vi "Trapezoidal SetAngle V2.vi"(0 "Current Angle":dbl, 5 "Desired Angle":dbl, 7 "\"dashboard values\"":T1) -> (1 "State":string, 2 "Completed?":bool, 3 "W reach in use":bool, 4 "Angular Velocity":dbl, 6 "Angular Acceleration":dbl, 8 "Current Angle":dbl, 10 "Time Completed":dbl, 13 "Reachable Velocity":dbl, 14 "Area":dbl, 15 "Times":cluster{"ta":dbl, "tc":dbl, "tf":dbl})   [LabVIEW 2015]
uses:
  TrapModeSetAngle.ctl
  Change Detect Double.vi
  Change Detect Int.vi
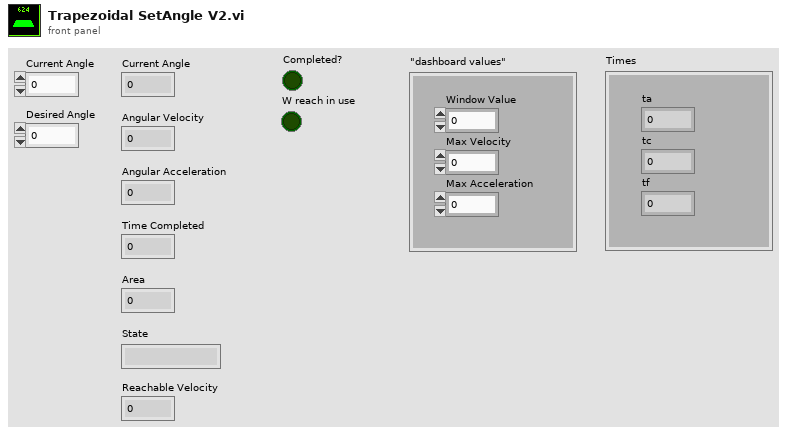
[diagram p1: front panel]
types:
  T1 = cluster{"Window Value":dbl, "Max Velocity":dbl, "Max Acceleration":dbl}
  T2 = typedef "TrapModeSetAngle.ctl" = enum16{"Accelerate", "Decelerate", "Cruz", "Finish"}
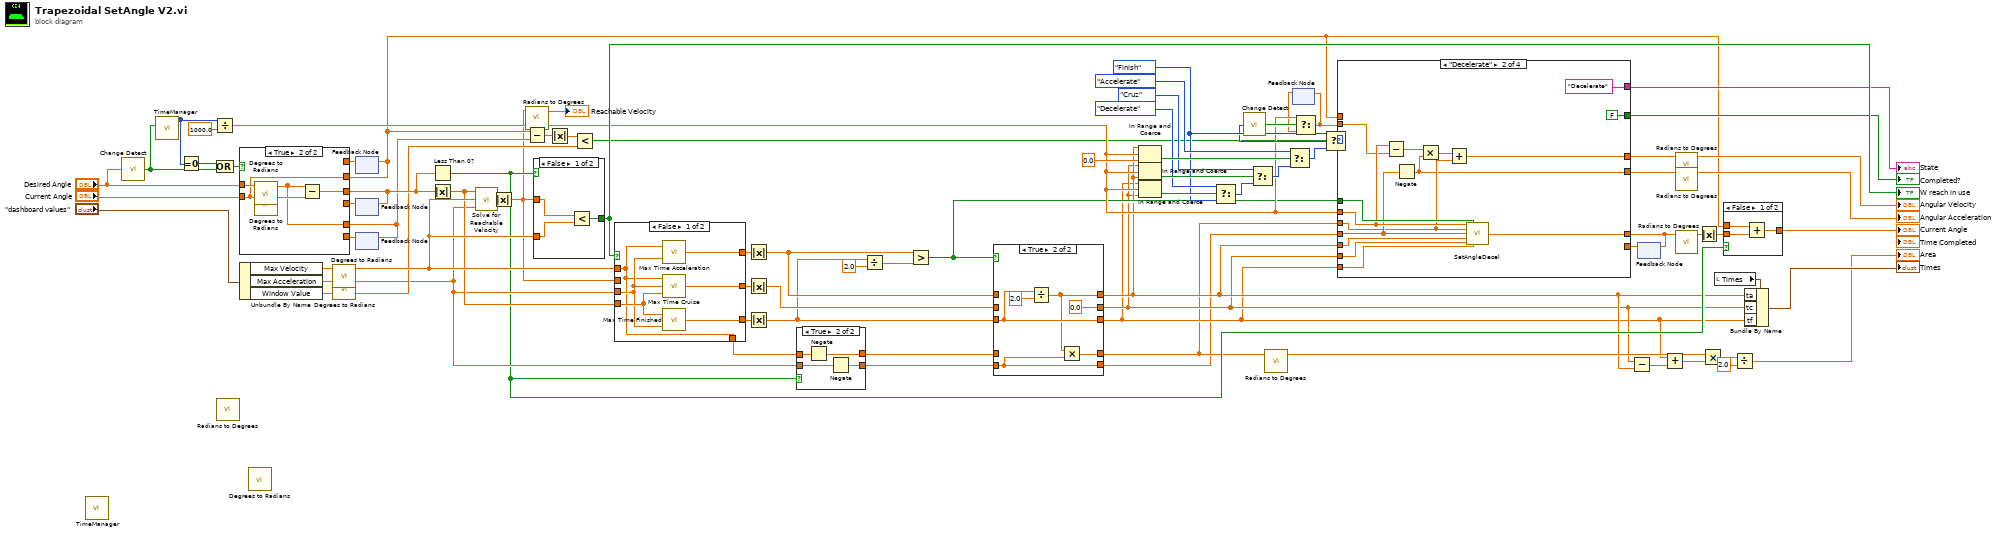
[diagram p0: block diagram]
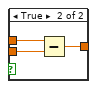
[diagram p3: hidden frame]
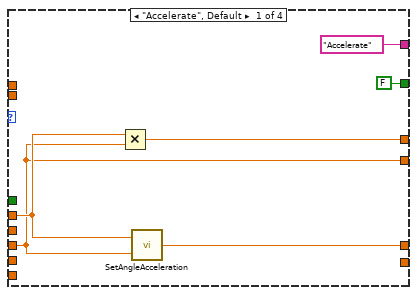
[diagram p5: hidden frame]
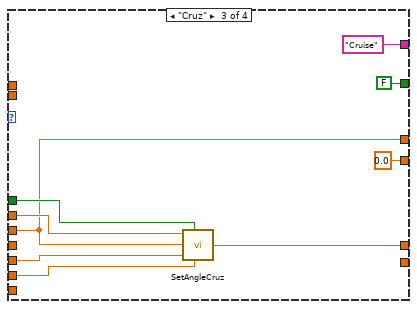
[diagram p6: hidden frame]
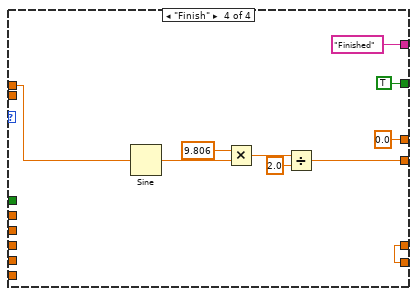
[diagram p7: hidden frame]
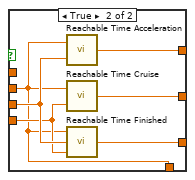
[diagram p8: hidden frame]
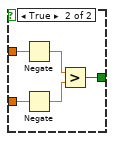
[diagram p9: hidden frame]
diagram:
  w54 = TrapModeSetAngle."Finish" ("Mode")
  n1 = call "TimeManager.vi"() -> ()  [unwired: 10 in, 2 out]
  n2 = call-poly "Change Detect.vi"("In"="Desired Angle") -> ("Changed?"=w75:bool)
  n3 = call "TimeManager.vi"("Reset?"=w75) -> ("Time Since Reset"=w65:u32)  [unwired: 9 in, 1 out]
  n4 = Equal To 0?(x=w65) -> (x = 0?=w74:bool)
  n5 = Divide(x=w65, y=1000.0) -> (x/y=w35:dbl)
  n6 = Compound Arithmetic op=OR(w74, w75) -> (w76:bool)
  n7 = call "Radians to Degrees.vi"() -> ()  [unwired: 5 in, 1 out]
  n8 = Unbundle By Name("\"dashboard values\"") -> ("Max Velocity"=w72:dbl, "Max Acceleration"=w71:dbl, "Window Value"=w49:dbl)
  n9 = call "Degrees to Radians.vi"() -> ()  [unwired: 5 in, 1 out]
  n10 = call "Degrees to Radians.vi"("Degrees IN"=w72) -> ("Radians OUT"=w70:dbl)  [unwired: 4 in]
  n11 = call "Degrees to Radians.vi"("Degrees IN"=w71) -> ("Radians OUT"=w47:dbl)  [unwired: 4 in]
  n12 = feedback #1() -> (w77:dbl)  [unwired: 1 in]
  n13 = feedback #2() -> (w78:dbl)  [unwired: 1 in]
  n14 = feedback #3() -> (w53:dbl)  [unwired: 1 in]
  n15 = case shown="True" w76 {
    tunnel: "Desired Angle" -> [_ w88]
    tunnel: "Current Angle" -> [_ w84]
    tunnel: [w83 w87] -> w73
    tunnel: w78 -> [w83 _]
    tunnel: [w82 w84] -> w24
    tunnel: w77 -> [w82 _]
    tunnel: [w81 w85] -> w52
    tunnel: w53 -> [w81 _]
    frame False {
    }
    frame True {
      n16 = call "Degrees to Radians.vi"("Degrees IN"=w88) -> ("Radians OUT"=w85:dbl)  [unwired: 4 in]
      n17 = call "Degrees to Radians.vi"("Degrees IN"=w84) -> ("Radians OUT"=w86:dbl)  [unwired: 4 in]
      n18 = Subtract(x=w85, y=w86) -> (x-y=w87:dbl)
    }
  }
  n19 = feedback-in #1(w24) -> ()
  n20 = feedback-in #2(w73) -> ()
  n21 = feedback-in #3(w52) -> ()
  n22 = Less Than 0?(x=w73) -> (x < 0?=w41:bool)
  n23 = Absolute Value(x=w73) -> (abs(x)=w69:dbl)
  n24 = call "Solve for Reachable Velocity.vi"("Max Acceleration"=w47, "Max Velocity"=w70, "Angular Displacement"=w69) -> ("Reachable Velocity"=w22:dbl)
  n25 = Absolute Value(x=w22) -> (abs(x)=w8:dbl)
  n26 = call "Radians to Degrees.vi"("Radians"=w8) -> ("Degrees"=→"Reachable Velocity":dbl)  [unwired: 4 in]
  n27 = Subtract(x=w24, y=w52) -> (x-y=w51:dbl)
  n28 = case shown="False" w41 {
    tunnel: w8 -> [w91 w96]
    tunnel: w70 -> [w90 w95]
    tunnel: [w89 w92] -> w42
    frame False {
      n29 = Less?(x=w91, y=w90) -> (x < y?=w89:bool)
    }
    frame True {
      n30 = Negate(x=w96) -> (-x=w94:dbl)
      n31 = Negate(x=w95) -> (-x=w93:dbl)
      n32 = Greater?(x=w94, y=w93) -> (0:w92:bool)
    }
  }
  "W reach in use" <- w42
  n33 = Absolute Value(x=w51) -> (abs(x)=w50:dbl)
  n34 = Less?(x=w50, y=w49) -> (x < y?=w25:bool)
  n35 = case shown="False" w42 {
    tunnel: w70 -> [w97 _]
    tunnel: w8 -> [_ w103]
    tunnel: w47 -> [w101 w108]
    tunnel: w69 -> [w102 w107]
    tunnel: [w100 w106] -> w18
    tunnel: [w99 w105] -> w19
    tunnel: [w98 w104] -> w20
    tunnel: [w97 w103] -> w48
    frame False {
      n36 = call "Max Time Acceleration.vi"("Max Acceleration"=w101, "Max Velocity"=w97) -> ("Max Time Acceleration"=w100:dbl)
      n37 = call "Max Time Cruise.vi"("Angle Displacement"=w102, "Max Acceleration"=w101, "Max Velocity"=w97) -> ("Max Time Cruise"=w99:dbl)
      n38 = call "Max Time Finished.vi"("Max Acceleration"=w101, "Angle Displacement"=w102) -> ("Max Time Finished"=w98:dbl)
    }
    frame True {
      n39 = call "Reachable Time Acceleration.vi"("Max Acceleration"=w108, "Reachable Angular Velocity"=w103) -> ("Reachable Time Acceleration"=w106:dbl)
      n40 = call "Reachable Time Cruise.vi"("Angle Displacement"=w107, "Reachable Angular Velocity"=w103) -> ("Reachable Time Cruise"=w105:dbl)
      n41 = call "Reachable Time Finished.vi"("Angle Displacement"=w107, "Max Acceleration"=w108, "Reachable Angular Velocity"=w103) -> ("Reachable Time Finished"=w104:dbl)
    }
  }
  n42 = Absolute Value(x=w18) -> (abs(x)=w11:dbl)
  n43 = Absolute Value(x=w19) -> (abs(x)=w10:dbl)
  n44 = Absolute Value(x=w20) -> (abs(x)=w9:dbl)
  n45 = case shown="True" w41 {
    tunnel: w48 -> [w110 w114]
    tunnel: w47 -> [w109 w113]
    tunnel: [w110 w112] -> w4
    tunnel: [w109 w111] -> w2
    frame False {
    }
    frame True {
      n46 = Negate(x=w114) -> (-x=w112:dbl)
      n47 = Negate(x=w113) -> (-x=w111:dbl)
    }
  }
  n48 = Divide(x=w9, y=2.0) -> (x/y=w45:dbl)
  n49 = Greater?(x=w11, y=w45) -> (0:w21:bool)
  n50 = case shown="True" w21 {
    tunnel: [w119 w122] -> w7
    tunnel: [w118 0.0 ("Reachable Time Cruise")] -> w6
    tunnel: [w117 w125] -> w5
    tunnel: w11 -> [w119 _]
    tunnel: w10 -> [w118 _]
    tunnel: w9 -> [w117 w125]
    tunnel: w4 -> [w116 _]
    tunnel: [w116 w121] -> w3
    tunnel: w2 -> [w115 w120]
    tunnel: [w115 w120] -> w1
    frame False {
    }
    frame True {
      n51 = Divide(x=w125, y=2.0) -> (x/y=w122:dbl)
      n52 = Multiply(x=w122, y=w120) -> (x*y=w121:dbl)
    }
  }
  n53 = In Range and Coerce(upper limit=w7, x=w35, lower limit=0.0) -> (In Range?=w63:bool)  [unwired: 1 out]
  n54 = In Range and Coerce(upper limit=w6, x=w35, lower limit=w7) -> (In Range?=w62:bool)  [unwired: 1 out]
  n55 = In Range and Coerce(upper limit=w5, x=w35, lower limit=w6) -> (In Range?=w60:bool)  [unwired: 1 out]
  n56 = Select(t=TrapModeSetAngle."Decelerate" ("Mode"), s=w60, f=w54) -> (s? t:f=w59:T2)
  n57 = Select(t=TrapModeSetAngle."Cruz" ("Mode"), s=w62, f=w59) -> (s? t:f=w61:T2)
  n58 = call "Radians to Degrees.vi"("Radians"=w3) -> ("Degrees"=w12:dbl)  [unwired: 4 in]
  n59 = Select(t=TrapModeSetAngle."Accelerate" ("Mode"), s=w63, f=w61) -> (s? t:f=w58:T2)
  n60 = feedback #4() -> (w34:dbl)  [unwired: 1 in]
  n61 = Select(t=w54, s=w25, f=w58) -> (s? t:f=w37:T2)
  n62 = call-poly "Change Detect.vi"("In"=w37) -> ("Changed?"=w36:bool)
  n63 = Select(t=w35, s=w36, f=w34) -> (s? t:f=w33:dbl)
  n64 = feedback-in #4(w33) -> ()
  n65 = Subtract(x=w6, y=w7) -> (x-y=w17:dbl)
  n66 = feedback #5() -> (w44:dbl)  [unwired: 1 in]
  n67 = case shown="\"Decelerate\"" w37 {
    tunnel: w7 -> [_ w145 w153 _]
    tunnel: w6 -> [_ w144 w152 _]
    tunnel: w5 -> [_ w143 _ _]
    tunnel: w1 -> [w127 w138 _ _]
    tunnel: w3 -> [_ w136 w150 _]
    tunnel: w35 -> [w130 w141 w155 _]
    tunnel: [w131 w146 w154 w165] -> w40
    tunnel: w21 -> [_ w142 w151 _]
    tunnel: w44 -> [_ _ _ w165]
    tunnel: w33 -> [_ w140 _ _]
    tunnel: [w129 w135 w150 0.0 ("Radians OUT")] -> w32
    tunnel: [w127 w134 0.0 w158] -> w31
    tunnel: ["Accelerate" "Decelerate" "Cruise" "Finished"] -> w30
    tunnel: [FALSE FALSE FALSE TRUE] -> w26
    tunnel: w24 -> [_ _ _ w156]
    frame "Accelerate", Default {
      n68 = Multiply(x=w130, y=w127) -> (x*y=w129:dbl)
      n69 = call "SetAngleAcceleration.vi"("Angular Acceleration"=w127, "Time Manager Output"=w130) -> ("Current Angle"=w131:dbl)
    }
    frame "Decelerate" {
      n70 = Subtract(x=w141, y=w140) -> (x-y=w139:dbl)
      n71 = Negate(x=w138) -> (-x=w134:dbl)
      n72 = Multiply(x=w139, y=w134) -> (x*y=w137:dbl)
      n73 = Add(x=w137, y=w136) -> (x+y=w135:dbl)
      n74 = call "SetAngleDecel.vi"("Time Manager Output"=w141, "ta > tf/2?"=w142, "Angular Velocity"=w136, "Angular Acceleration"=w138, "Time Acceleration"=w145, "Time Cruise"=w144, "Time Finished"=w143) -> ("CurrentAngle"=w146:dbl)  [unwired: 8 in]
    }
    frame "Cruz" {
      n75 = call "SetAngleCruz.vi"("Time Manager Output"=w155, "ta > tf/2?"=w151, "Angular Velocity"=w150, "Time Acceleration"=w153, "Time Cruise"=w152) -> ("Current Angle"=w154:dbl)
    }
    frame "Finish" {
      n76 = Sine(x=w156) -> (sin(x)=w161:dbl)
      n77 = Multiply(x=9.806, y=w161) -> (x*y=w160:dbl)
      n78 = Divide(x=w160, y=2.0) -> (x/y=w158:dbl)
    }
  }
  "Completed?" <- w26
  "State" <- w30
  n79 = feedback-in #5(w40) -> ()
  n80 = Add(x=w5, y=w17) -> (x+y=w16:dbl)
  n81 = call "Radians to Degrees.vi"("Radians"=w32) -> ("Degrees"=→"Angular Velocity":dbl)  [unwired: 4 in]
  n82 = call "Radians to Degrees.vi"("Radians"=w31) -> ("Degrees"=→"Angular Acceleration":dbl)  [unwired: 4 in]
  n83 = call "Radians to Degrees.vi"("Radians"=w40) -> ("Degrees"=w39:dbl)  [unwired: 4 in]
  n84 = Absolute Value(x=w39) -> (abs(x)=w38:dbl)
  n85 = Multiply(x=w12, y=w16) -> (x*y=w15:dbl)
  n86 = local read "Times"() -> (w68:cluster{"ta":dbl, "tc":dbl, "tf":dbl})
  n87 = case shown="False" w41 {
    tunnel: w38 -> [w168 w171]
    tunnel: [w167 w170] -> w43
    tunnel: w24 -> [w166 w169]
    frame False {
      n88 = Add(x=w166, y=w168) -> (x+y=w167:dbl)
    }
    frame True {
      n89 = Subtract(x=w169, y=w171) -> (x-y=w170:dbl)
    }
  }
  "Current Angle" <- w43
  n90 = Divide(x=w15, y=2.0) -> (x/y=→"Area":dbl)
  n91 = Bundle By Name(cluster=w68, "ta"=w7, "tc"=w6, "tf"=w5) -> (→"Times":cluster{"ta":dbl, "tc":dbl, "tf":dbl})
